vi "Initialise.vi"(8 "error in (no error)":errorcluster, 9 "EEPROM":refnum<class "EEPROM.lvclass">, 10 "RAM":refnum<class "RAM.lvclass">, 11 "Memory Map":refnum<class "Memory Map.lvclass">) -> (0 "error out":errorcluster, 3 "Clock Generator":refnum<class "IO.lvclass">)   [LabVIEW 2021, in "IO.lvclass"]
uses:
  IO.lvclass
  Memory Map/Memory Map.lvclass
  RAM/RAM.lvclass
  EEPROM/EEPROM.lvclass
  IO.lvclass/IO.ctl
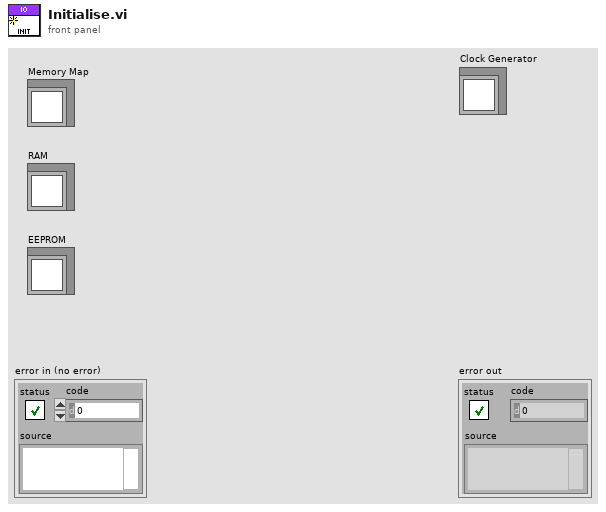
[diagram p1: front panel]
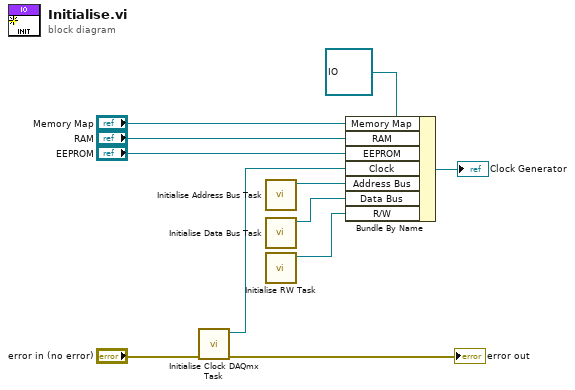
[diagram p0: block diagram]
diagram:
  n1 = call "Initialise Clock DAQmx Task.vi"("error in"="error in (no error)") -> ("error out"=→"error out":errorcluster, "task out"=w11:refnum<k21>)  [unwired: 9 in]
  n2 = call "Initialise Address Bus Task.vi"() -> ("Address Bus"=w6:refnum<k21>)  [unwired: 10 in, 1 out]
  n3 = call "Initialise Data Bus Task.vi"() -> ("Data Bus"=w5:refnum<k21>)  [unwired: 10 in, 1 out]
  n4 = call "Initialise RW Task.vi"() -> ("R/W"=w4:refnum<k21>)  [unwired: 10 in, 1 out]
  n5 = Bundle By Name(cluster=refnum<class "IO.lvclass"> refnum ("Clock Generator out"), "Memory Map"="Memory Map", "RAM"="RAM", "EEPROM"="EEPROM", "Clock"=w11, "Address Bus"=w6, "Data Bus"=w5, "R/W"=w4) -> (→"Clock Generator":refnum<class "IO.lvclass">)
